vi "Page_Source_Can_Add_to_Top.vi"(6 "Project Refnum":refnum<vi>, 8 "error in (no error)":errorcluster, 10 "AB_Source in":refnum<class "AB_Source.lvclass">, 11 "AB_Build in":refnum<class "AB_Build.lvclass">) -> (0 "error out":errorcluster, 1 "message":string, 2 "canAddToTop":bool, 3 "AB_Build out":refnum<class "AB_Build.lvclass">)   [LabVIEW 2020, in "AB_Build.lvclass"]
uses:
  <vilib>/AppBuilder/AB_Classes/Build/AB_Build.lvclass
  <vilib>/AppBuilder/AB_Classes/Source/AB_Source.lvclass
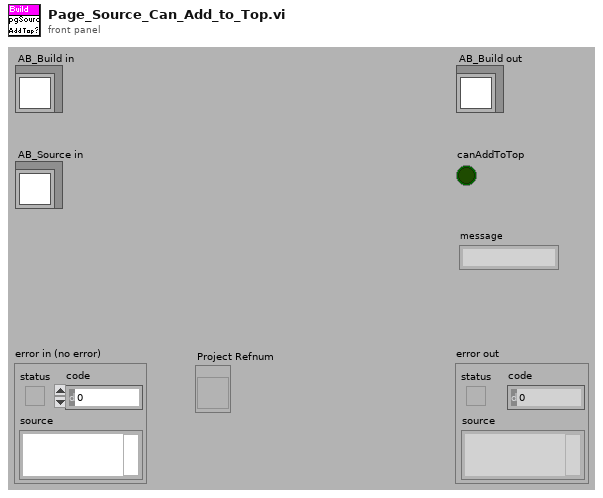
[diagram p1: front panel]
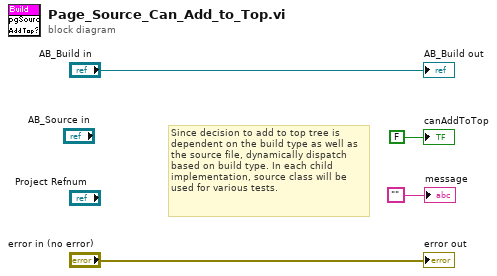
[diagram p0: block diagram]
diagram:
  # "Since decision to add to top tree is dependent on the build type as well as the source file, dynamically dispatch based on build type. In each child implementation, source class will be used for various tests."
  "error out" <- "error in (no error)"
  "AB_Build out" <- "AB_Build in"
  "canAddToTop" <- FALSE ("canAddToTop")
  "message" <- ""
